vi "LcWebView_example_2.vi"() -> ()   [LabVIEW 2019, in "LcWebView.lvclass"]
uses:
  LcWebView.lvclass
  C:/Projects/WebView2/LcWebView/data/Microsoft.Web.WebView2.WinForms.dll
panel:
  out "Javascript result":string
  out "HTML content":string
  out "Initialise Loops":i32
  out "Status Message":string
  out "Status":i32(ring) items=["Created", "WaitingForActivation", "WaitingToRun", "Running", "WaitingForChildrenToComplete", "RanToCompletion", "Canceled", "Faulted"]
  out "Error Out":errorcluster
  in  "stop":bool
  in  "Web":refnum<k24>(container)
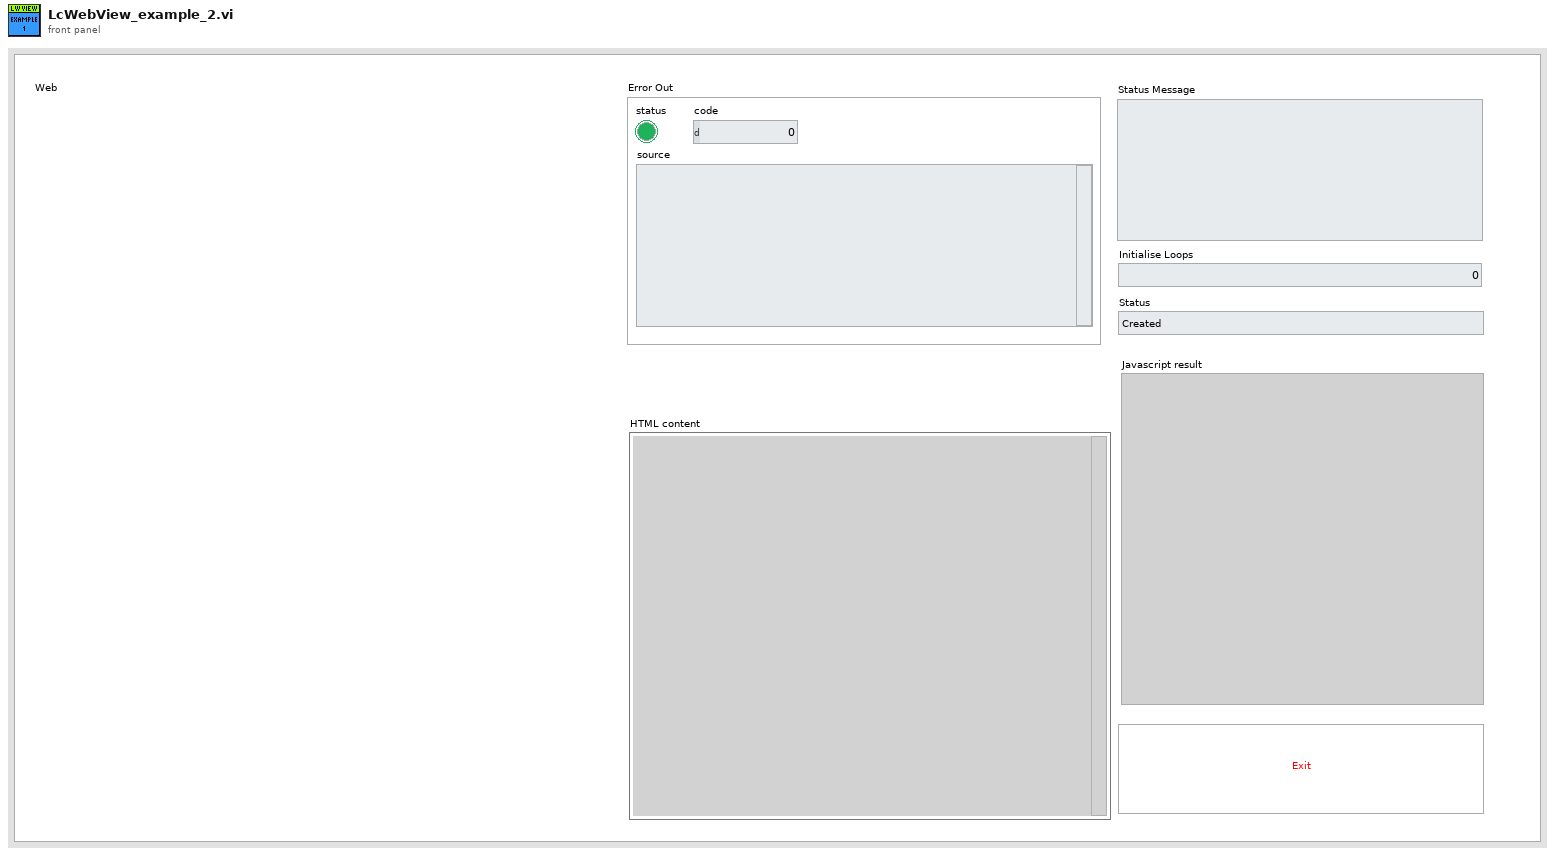
[diagram p1: front panel]
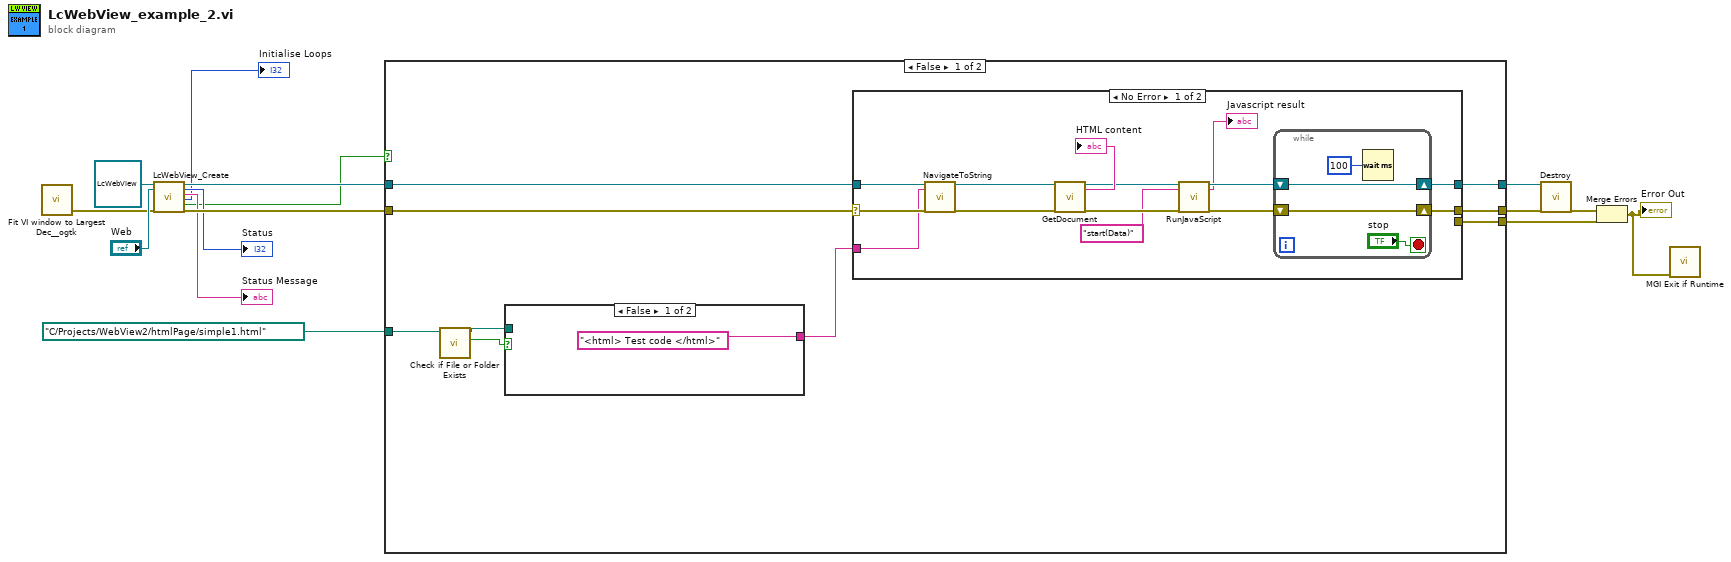
[diagram p0: block diagram]
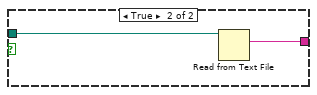
[diagram p2: hidden frame]
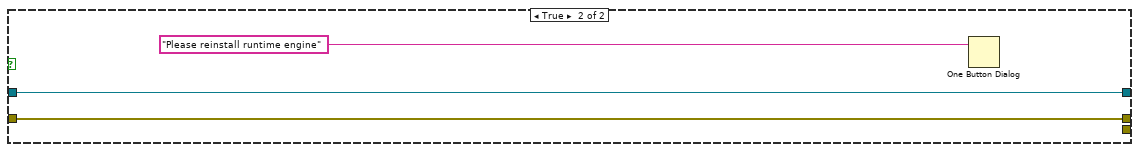
[diagram p4: hidden frame]
diagram:
  n1 = call "Fit VI window to Largest Dec__ogtk.vi"() -> ("error out"=w3:errorcluster)  [unwired: 6 in, 1 out]
  n2 = call "LcWebView_Create.vi"("reference in"=refnum<class "LcWebView.lvclass"> refnum, "Webview container"="Web", "Error In"=w3) -> ("reference out"=w13:refnum<class "LcWebView.lvclass">, "Status"=→"Status":i32, "Status Message"=→"Status Message":string, "Initialise Loops"=→"Initialise Loops":i32, "Reinstall Runtime"=w4:bool, "Error Out"=w12:errorcluster)  [unwired: 9 in, 2 out]
  n3 = case shown="False" w4 {
    tunnel: w13 -> [w24 w50]
    tunnel: w12 -> [w23 w49]
    tunnel: [w22 w50] -> w11
    tunnel: [w21 w49] -> w10
    tunnel: [w20 _] -> w5
    tunnel: path "C:/Projects/WebView2/htmlPage/simple1.html" ("DLLs path In") -> [w19 _]
    frame False {
      n4 = call <vilib>:"Check if File or Folder Exists.vi"("path"=w19) -> ("file or folder exists?"=w16:bool, "dup path"=w18:path)  [unwired: 8 in, 1 out]
      n5 = case shown="False" w16 {
        tunnel: w18 -> [_ w27]
        tunnel: ["<html> Test code </html>" ("HTML Content") w26] -> w17
        frame False {
        }
        frame True {
          n6 = Read from Text File(file (use dialog)=w27) -> (text=w26:string)  [unwired: 3 in, 3 out]
        }
      }
      n7 = case shown="No Error" w23 {
        selector: w23 -> [w29 w46]
        tunnel: w24 -> [w30 w47]
        tunnel: [w41 w47] -> w22
        tunnel: [w40 _] -> w21
        tunnel: [_ w46] -> w20
        tunnel: w17 -> [w28 _]
        frame No Error {
          n8 = call-dynamic "NavigateToString.vi"("reference in"=w30, "HTML Content"=w28, "Error In"=w29) -> ("reference out"=w32:refnum<class "LcWebView.lvclass">, "Error Out"=w31:errorcluster)  [unwired: 14 in, 1 out]
          n9 = call-dynamic "GetDocument.vi"("reference in"=w32, "Error In"=w31) -> ("reference out"=w38:refnum<class "LcWebView.lvclass">, "Result"=→"HTML content":string, "Error Out"=w37:errorcluster)  [unwired: 15 in]
          n10 = call-dynamic "RunJavaScript.vi"("reference in"=w38, "Java Script Function"="start(Data)", "Error In"=w37) -> ("reference out"=w36:refnum<class "LcWebView.lvclass">, "Result"=→"Javascript result":string, "Error Out"=w35:errorcluster)  [unwired: 13 in, 1 out]
          n11 = while {
            shift-right: [w44] -> w41
            shift-left: w36 -> [w44]
            shift-right: [w43] -> w40
            shift-left: w35 -> [w43]
            stop <- "stop" stop-if-true
            n12 = Wait (ms)(milliseconds to wait=u32 100) -> ()  [unwired: 1 out]
          }
        }
        frame Error {
        }
      }
    }
    frame True {
      n13 = One Button Dialog(message="Please reinstall runtime engine") -> ()  [unwired: 1 in, 1 out]
    }
  }
  n14 = call-dynamic "Destroy.vi"("reference in"=w11, "Error In"=w10) -> ("Error Out"=w9:errorcluster)  [unwired: 16 in, 1 out]
  n15 = Merge Errors(w9, w5) -> (w2:errorcluster)
  "Error Out" <- w2
  n16 = call "MGI Exit if Runtime.vi"("Error In (Dependency Only)"=w2) -> ()  [unwired: 11 in]
